vi "Slope Calibration Inputs to XML.vi"() -> (0 "XML Data":string)   [LabVIEW 2013]
uses:
  Types/Slope Calibration Inputs.ctl
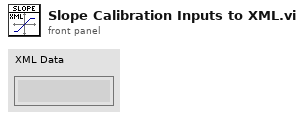
[diagram p1: front panel]
types:
  T1 = typedef "Slope Calibration Inputs.ctl" = cluster{"Number of Samples":dbl, "Ramp Rate":dbl, "Z Scan Size":dbl, "Version":string}
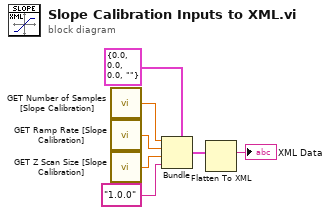
[diagram p0: block diagram]
diagram:
  n1 = call "GET Number of Samples [Slope Calibration].vi"() -> ("Number of Samples"=w3:dbl)
  n2 = call "GET Ramp Rate [Slope Calibration].vi"() -> ("Ramp Rate"=w5:dbl)
  n3 = call "GET Z Scan Size [Slope Calibration].vi"() -> ("Z Scan Size"=w4:dbl)
  n4 = Bundle(cluster=T1 {"Number of Samples"=0.0, "Ramp Rate"=0.0, "Z Scan Size"=0.0, "Version"=""} ("Slope Calibration Inputs"), "Number of Samples"=w3, "Ramp Rate"=w5, "Z Scan Size"=w4, "Version"="1.0.0") -> (w6:T1)
  n5 = Flatten To XML(anything=w6) -> (xml string=→"XML Data":string)
